vi "forma.vi"(5 "Input param":T1, 7 "GradFilePath":path caption="Градуировкиа:") -> ()   [LabVIEW 2010]
uses:
  <vilib>/Utility/config.llb/Read Key (Path).vi
  <vilib>/Utility/config.llb/Read Key (I32).vi
  <vilib>/Utility/config.llb/Write Key (I32).vi
  <vilib>/Utility/config.llb/NI_LVConfig.lvlib
panel:
  in  "Tab Control":T2(tab)
  in  "Channels":bool[](array[boolean]) caption="Каналы"
  in  "Sensors":string(combo) caption="Датчики:"
  in  "Conditions":string(combo) caption="Напряжение кВ:"
  in  "TesterName":string(combo) caption="Испытатель:"
  in  "Description":string(combo) caption="Измерение ЧР в:"
  out "ADCNum":string="Корона-20 № 11 АЦП 496" caption="Измеритель:"
  out "RepDate":string="2:23:15 24.11.2014" caption="Дата:"
  out "ObjName":string="Трансформатор № 1089-23" caption="Объект:"
  in  "RepNum":string="000012-03-2014.11.24" caption="Протокол номер:"
  in  "Concl":string="Заключение: " caption="Заключение"
  in  "CreateRepBtn":bool caption="Создать отчет"
  in  "ExitBtn":bool caption="Выйти"
  out "N(Q)":cluster{"x0":dbl, "dx":dbl, "y":sgl[][]}(graph) caption="Гистограмма N (Q)"
  out "Q(fi)":cluster{"x0":dbl, "dx":dbl, "y":sgl[][]}(graph) caption="Распределение @ ЧР по Фазе"
  out "Зависимость токов ЧР от I(R)":cluster{"x0":dbl, "dx":dbl, "y":sgl[][]}(graph) caption="Зависимость токов ЧР от коэффициента стационарности R"
  out "Q(R)":cluster{"x0":dbl, "dx":dbl, "y":sgl[][]}(graph) caption="Зависимость Q ЧР от коэффициента стационарности R"
  # "К1               К2               К3                К4"
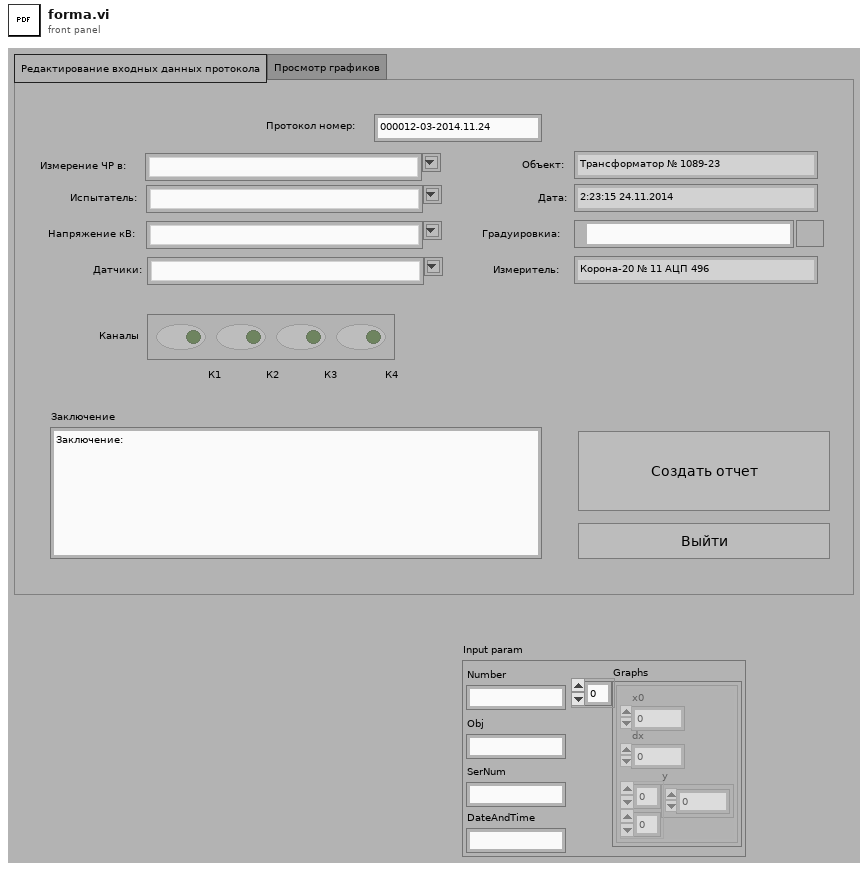
[diagram p1: front panel]
types:
  T1 = cluster{"Number":string, "Obj":string, "SerNum":string, "Graphs":cluster{"x0":dbl, "dx":dbl, "y":sgl[][]}[], "DateAndTime":string}
  T2 = enum32{"Редактирование входных данных протокола", "Просмотр графиков"}
  T3 = typedef "NI_LVConfig.lvlib/Config Data RefNum.ctl" = refnum<k1>
  T4 = cluster{"RepNum":string, "Description":string, "TesterName":string, "Conditions":string, "Sensors":string, "ObjName":string, string, string, "ADCNum":string, "Concl":string, "date/time string":string, "Channels":bool[], sgl[][]}
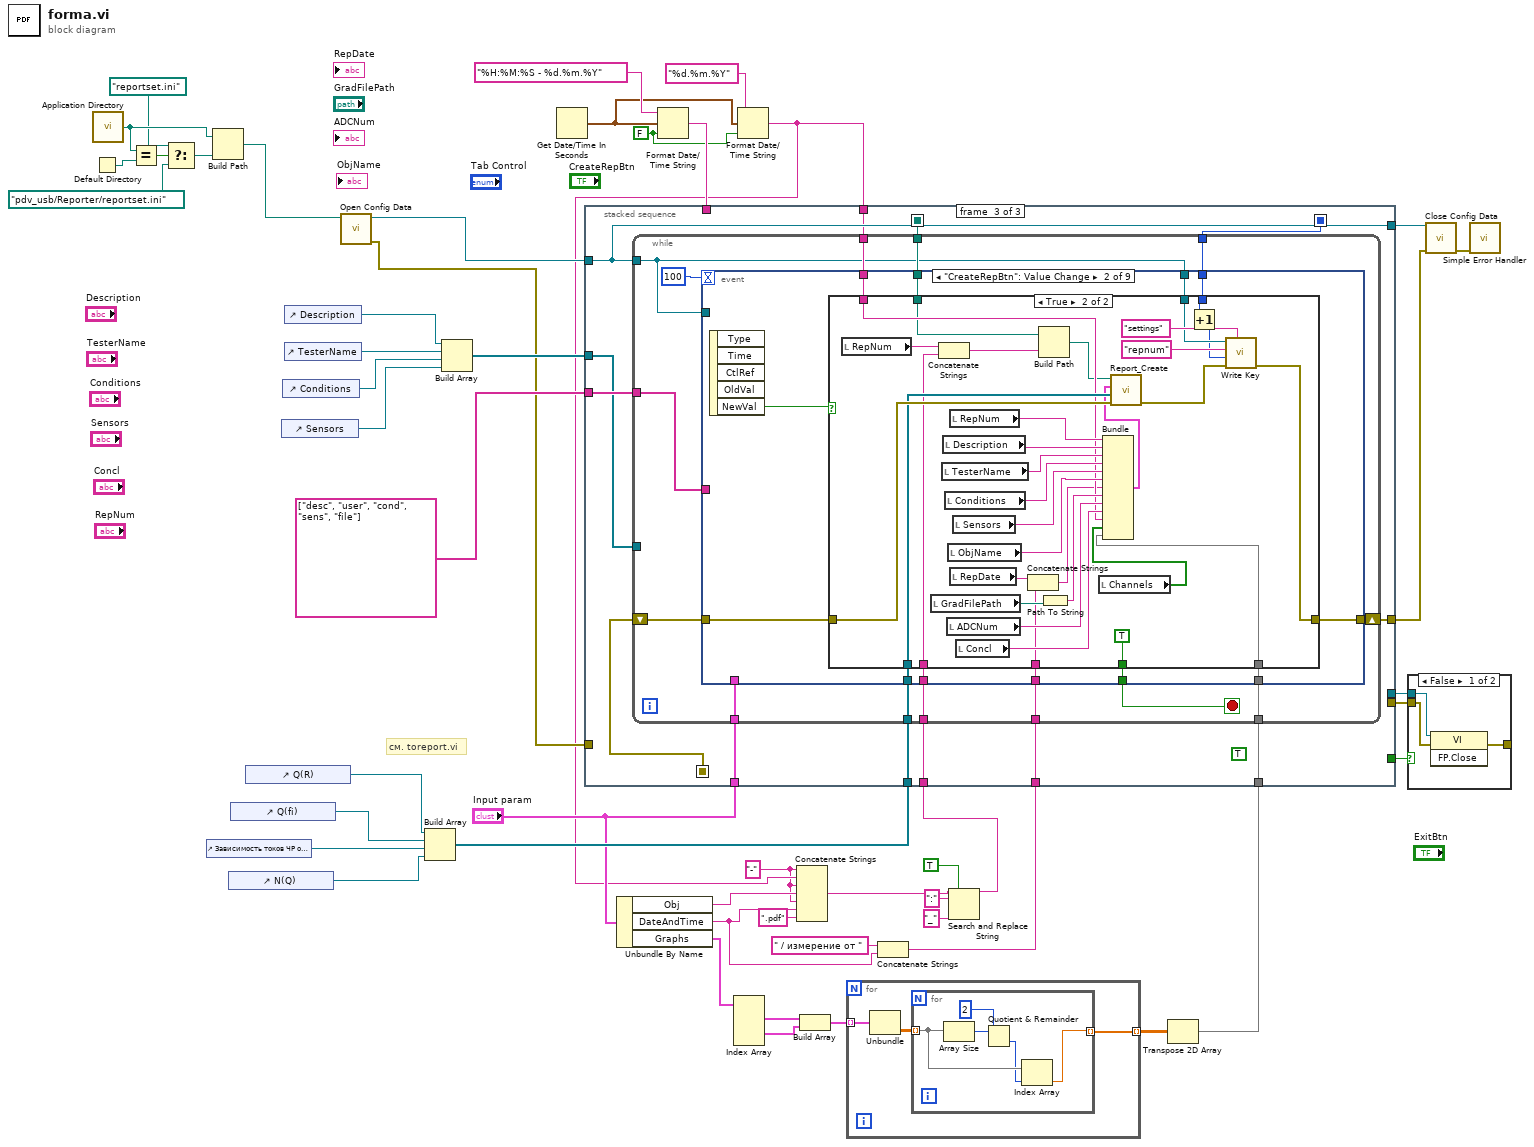
[diagram p0: block diagram]
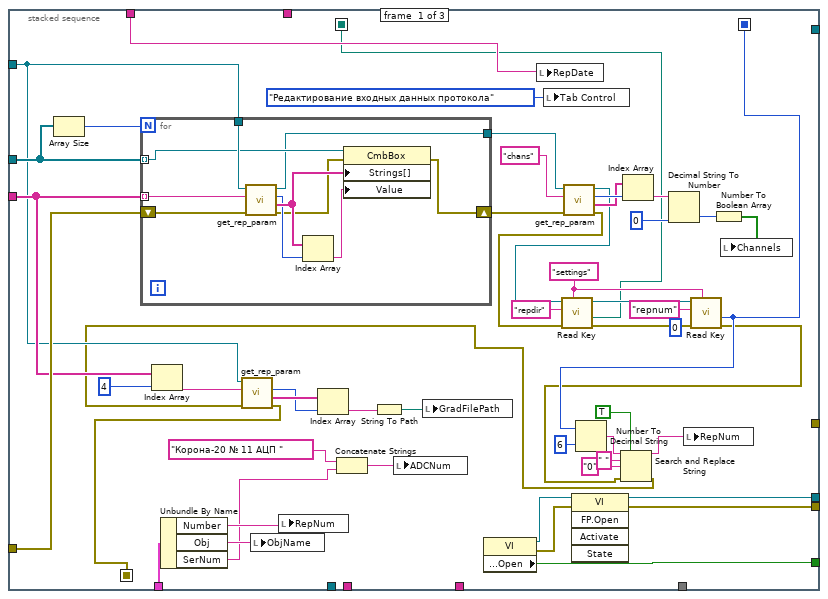
[diagram p3: hidden frame]
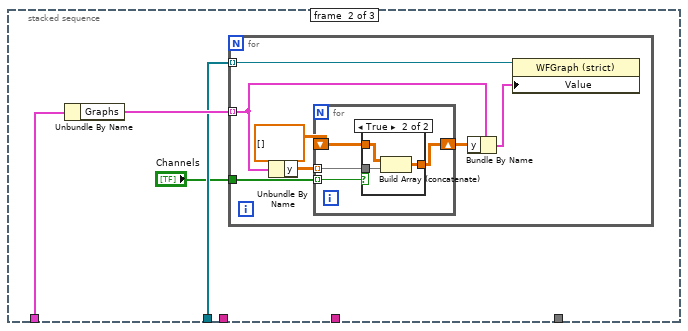
[diagram p4: hidden frame]
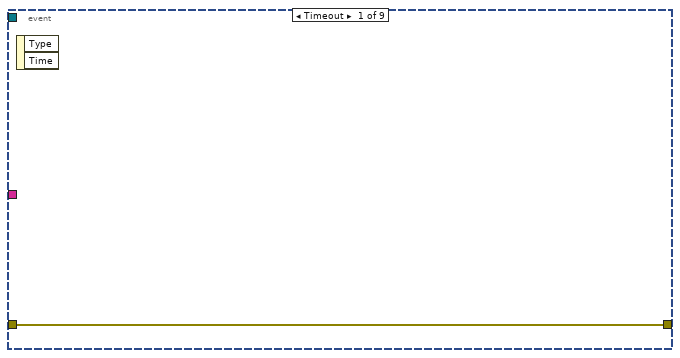
[diagram p6: hidden frame]
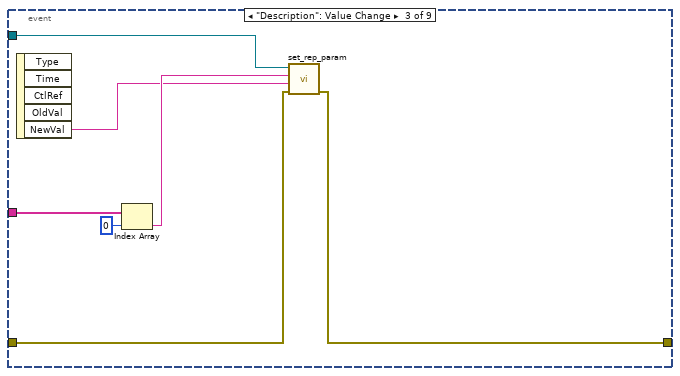
[diagram p8: hidden frame]
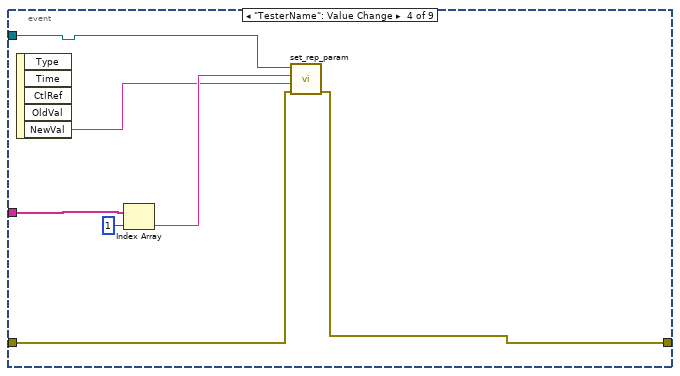
[diagram p9: hidden frame]
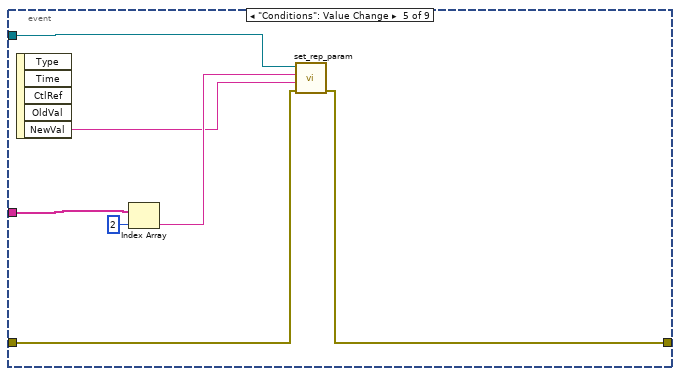
[diagram p10: hidden frame]
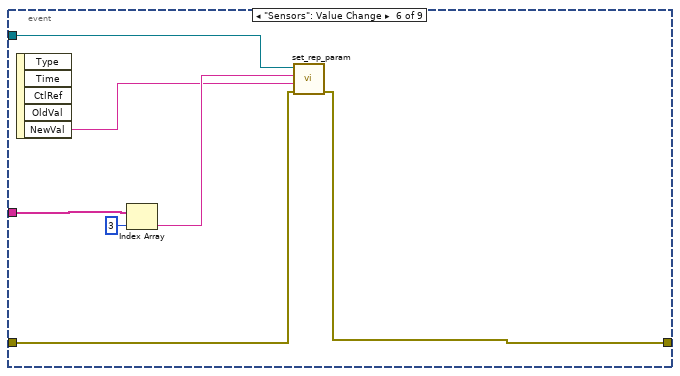
[diagram p11: hidden frame]
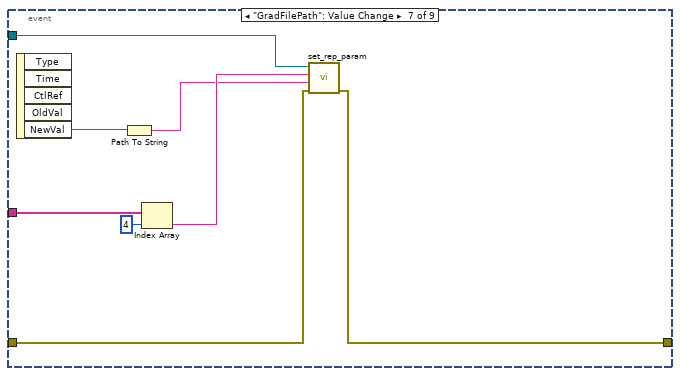
[diagram p12: hidden frame]
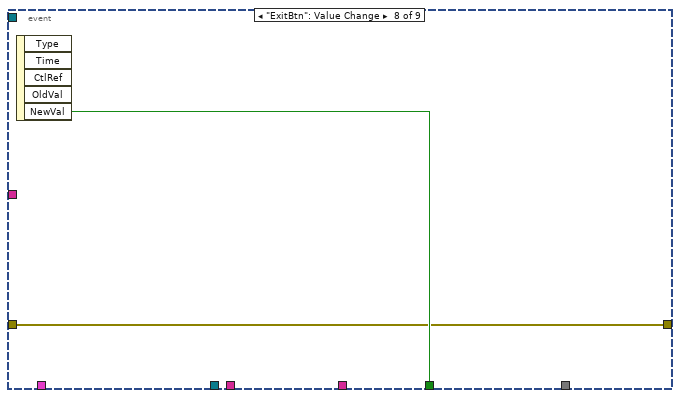
[diagram p13: hidden frame]
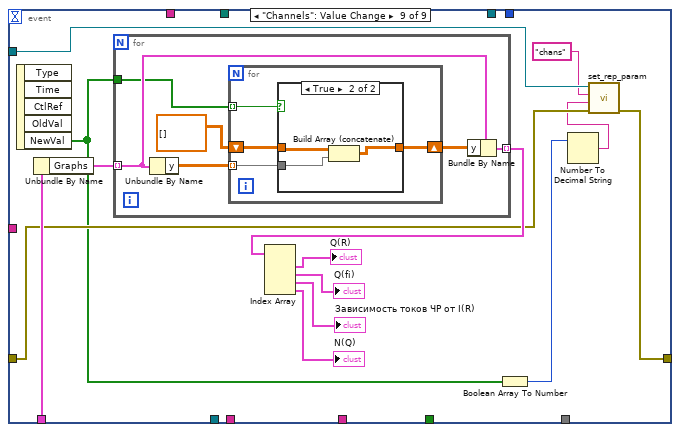
[diagram p14: hidden frame]
diagram:
  w16 = "-" ("string")
  w19 = FALSE ("UTC format")
  # "см. toreport.vi"
  n1 = Default Directory() -> (w28:path)
  n2 = call <vilib>:"Application Directory.vi"() -> ("Application Directory"=w27:path)
  n3 = Equal?(x=w27, y=w28) -> (x = y?=w26:bool)
  n4 = Select(t=path "reportset.ini" ("configuration file path"), s=w26, f=path "pdv_usb/Reporter/reportset.ini" ("configuration file path")) -> (s? t:f=w24:path)
  n5 = control-ref of="Зависимость токов ЧР от I(R)"() -> (w39:refnum<vi>)
  n6 = Build Path(base path=w27, name or relative path=w24) -> (appended path=w29:path)
  n7 = control-ref of="N(Q)"() -> (w38:refnum<vi>)
  n8 = control-ref of="Q(fi)"() -> (w40:refnum<vi>)
  n9 = control-ref of="Q(R)"() -> (w37:refnum<vi>)
  n10 = control-ref of="Sensors"() -> (w47:refnum<vi>)
  n11 = control-ref of="Conditions"() -> (w48:refnum<vi>)
  n12 = control-ref of="Description"() -> (w50:refnum<vi>)
  n13 = control-ref of="TesterName"() -> (w49:refnum<vi>)
  n14 = call <vilib>:"Open Config Data.vi"("configuration file path"=w29) -> ("error out"=w43:errorcluster, "refnum"=w44:T3)  [unwired: 8 in, 1 out]
  n15 = Build Array(w37, w40, w39, w38) -> (w36:refnum<vi>[])
  n16 = Build Array(w50, w49, w48, w47) -> (w46:refnum<vi>[])
  n17 = Get Date/Time In Seconds() -> (seconds since 1Jan1904=w20:timestamp)
  n18 = Unbundle By Name("Input param") -> ("Obj"=w17:string, "DateAndTime"=w13:string, "Graphs"=w6:cluster{"x0":dbl, "dx":dbl, "y":sgl[][]}[])
  n19 = Format Date/Time String(time format string (%c)="%H:%M:%S - %d.%m.%Y", seconds (now)=w20, UTC format=w19) -> (date/time string=w34:string)
  n20 = Index Array(array=w6) -> (element #1=w5:cluster{"x0":dbl, "dx":dbl, "y":sgl[][]}, element #3=w4:cluster{"x0":dbl, "dx":dbl, "y":sgl[][]})  [unwired: 4 in, 2 out]
  n21 = Format Date/Time String(time format string (%c)="%d.%m.%Y", seconds (now)=w20, UTC format=w19) -> (date/time string=w18:string)
  n22 = Concatenate Strings(w16, w18, w16, w17, w16, w13, ".pdf" ("string")) -> (w10:string)
  n23 = Build Array(w5, w4) -> (w3:cluster{"x0":dbl, "dx":dbl, "y":sgl[][]}[])
  n24 = for {
    tunnel: w3 -> [w53] mode=indexing
    tunnel: [w51] -> w2 mode=indexing
    n25 = Unbundle(w53) -> ("y"=w52:sgl[][])  [unwired: 2 out]
    n26 = for {
      tunnel: w52 -> [w56] mode=indexing
      tunnel: [w54] -> w51 mode=indexing
      n27 = Array Size(array=w56) -> (size(s)=w58:i32)
      n28 = Quotient & Remainder(x=w58, y=2) -> (floor(x/y)=w55:i32)  [unwired: 1 out]
      n29 = Index Array(array=w56, index=w55) -> (element=w54:sgl)
    }
  }
  n30 = Concatenate Strings(" / измерение от " ("string"), w13) -> (w12:string)
  n31 = Search and Replace String(replace all?=TRUE ("replace all? (F)"), input string=w10, search string=":", replace string="_" ("replace string (\"\")")) -> (result string=w9:string)  [unwired: 4 in, 3 out]
  n32 = Transpose 2D Array(2D array=w2) -> (transposed array=w1:sgl[][])
  n33 = stacked-sequence {
    seq-local: [w107 _ _] -> [_ _ w152]
    seq-local: [w59 _ _] -> [_ _ w143]
    seq-local: [w69 _ _] -> [_ _ w142]
    tunnel: w46 -> [w108 _ w149]
    tunnel: string[] ["desc", "user", "cond", "sens", "file"] -> [w105 _ w150]
    tunnel: w44 -> [w104 _ w148]
    tunnel: w43 -> [w110 _ _]
    tunnel: [_ _ w151] -> w41
    tunnel: [_ _ w148] -> w42
    tunnel: w36 -> [_ w122 w147]
    tunnel: w34 -> [w96 _ _]
    tunnel: "Input param" -> [w95 w124 w146]
    tunnel: [w89 _ _] -> w33
    tunnel: [w68 _ _] -> w32
    tunnel: [w88 _ _] -> w30
    tunnel: w18 -> [_ _ w145]
    tunnel: w9 -> [_ _ w144]
    tunnel: w12 -> [_ _ w141]
    tunnel: w1 -> [_ _ w140]
    frame #0 {
      w74 = "settings" ("section")
      n34 = Array Size(array=w108) -> (size(s)=w109:i32)
      n35 = for {
        N: w109 -> [_]
        tunnel: w108 -> [w117] mode=indexing
        tunnel: w105 -> [w119] mode=indexing
        tunnel: w104 -> [w120]
        shift-right: [w112] -> w85
        shift-left: w110 -> [w118]
        tunnel: [w111] -> w87
        n36 = call "get_rep_param.vi"("error in (no error)"=w118, "param_name"=w119, "refnum"=w120) -> ("error out"=w113:errorcluster, "list"=w116:string[], "default"=w115:i32, "refnum out"=w111:T3)  [unwired: 1 in]
        n37 = Index Array(array=w116, index=w115) -> (element=w114:string)
        n38 = property class="CmbBox"(reference=w117, error in=w113, "Strings[]"=w116, "Value"=w114) -> (error out=w112:errorcluster)  [unwired: 1 out]
      }
      n39 = Index Array(array=w105, index=4) -> (element=w103:string)
      n40 = Unbundle By Name(w95) -> ("Number"=w94:string, "Obj"=w93:string, "SerNum"=w92:string)
      n41 = local write "ObjName"(w93) -> ()
      n42 = local write "RepNum"(w94) -> ()
      n43 = Concatenate Strings("Корона-20 № 11 АЦП " ("time format string (%c)"), w92) -> (w97:string)
      n44 = local write "ADCNum"(w97) -> ()
      n45 = property class="VI"() -> (reference out=w91:refnum<vi>, error out=w90:errorcluster, "Front Panel.Open"=w89:bool)  [unwired: 2 in]
      n46 = local write "RepDate"(w96) -> ()
      n47 = local write "Tab Control"(T2."Редактирование входных данных протокола" ("Tab Control")) -> ()
      n48 = call "get_rep_param.vi"("error in (no error)"=w85, "param_name"="chans", "refnum"=w87) -> ("error out"=w78:errorcluster, "list"=w83:string[], "default"=w84:i32, "refnum out"=w76:T3)  [unwired: 1 in]
      n49 = call-poly <vilib>:"Read Key.vi"("section"=w74, "error in (no error)"=w78, "key"="repdir", "refnum"=w76) -> ("error out"=w77:errorcluster, "value"=w59:path, "refnum out"=w75:T3)  [unwired: 4 in, 1 out]
      n50 = invoke class="VI" method="FP.Open"(reference=w91, error in=w90) -> (reference out=w88:refnum<vi>, error out=w68:errorcluster)  [unwired: 3 in, 3 out]
      n51 = Index Array(array=w83, index=w84) -> (element=w82:string)
      n52 = Decimal String To Number(string=w82, default (0L)=u8 0) -> (number=w80:u8)  [unwired: 1 in, 1 out]
      n53 = call-poly <vilib>:"Read Key.vi"("section"=w74, "error in (no error)"=w77, "default value"=0, "key"="repnum", "refnum"=w75) -> ("error out"=w61:errorcluster, "value"=w69:i32)  [unwired: 3 in, 2 out]
      n54 = Number To Decimal String(number=w69, width (-)=i16 6) -> (decimal integer string=w65:string)
      n55 = Search and Replace String(replace all?=TRUE ("replace all? (F)"), input string=w65, search string=" ", replace string="0" ("replace string (\"\")"), error in=w61) -> (result string=w64:string, error out=w60:errorcluster)  [unwired: 3 in, 2 out]
      n56 = call "get_rep_param.vi"("error in (no error)"=w60, "param_name"=w103, "refnum"=w104) -> ("error out"=w107:errorcluster, "list"=w102:string[], "default"=w101:i32)  [unwired: 1 in, 1 out]
      n57 = Index Array(array=w102, index=w101) -> (element=w100:string)
      n58 = String To Path(string=w100) -> (path=w99:path)
      n59 = local write "GradFilePath"(w99) -> ()
      n60 = local write "RepNum"(w64) -> ()
      n61 = Number To Boolean Array(number=w80) -> (Boolean array=w79:bool[])
      n62 = local write "Channels"(w79) -> ()
    }
    frame #1 {
      n63 = Unbundle By Name(w124) -> ("Graphs"=w123:cluster{"x0":dbl, "dx":dbl, "y":sgl[][]}[])
      n64 = for {
        tunnel: w123 -> [w127] mode=indexing
        tunnel: w122 -> [w131] mode=indexing
        tunnel: "Channels" -> [w130]
        n65 = Unbundle By Name(w127) -> ("y"=w129:sgl[][])
        n66 = for {
          tunnel: w130 -> [w132] mode=indexing
          tunnel: w129 -> [w135] mode=indexing
          shift-right: [w134] -> w125
          shift-left: sgl[][] [] -> [w133]
          n67 = case shown="True" w132 {
            tunnel: w135 -> [_ w139]
            tunnel: [w136 w138] -> w134
            tunnel: w133 -> [w136 w137]
            frame False {
            }
            frame True {
              n68 = Build Array (concatenate)(w137, w139) -> (w138:sgl[][])
            }
          }
        }
        n69 = Bundle By Name(cluster=w127, "y"=w125) -> (w126:cluster{"x0":dbl, "dx":dbl, "y":sgl[][]})
        n70 = property class="WFGraph (strict)"(reference=w131, "Value"=w126) -> ()  [unwired: 1 in, 2 out]
      }
    }
    frame #2 {
      (unwired) TRUE
      n71 = while {
        shift-right: [w164] -> w151
        shift-left: w152 -> [w165]
        tunnel: w148 -> [w156]
        tunnel: w150 -> [w163]
        tunnel: w149 -> [_]
        tunnel: w147 -> [w161]
        tunnel: w146 -> [w160]
        tunnel: w145 -> [w159]
        tunnel: w144 -> [w158]
        tunnel: w143 -> [w157]
        tunnel: w142 -> [w155]
        tunnel: w141 -> [w154]
        tunnel: w140 -> [w153]
        stop <- w166 stop-if-true
        n72 = event shown="[1] \"CreateRepBtn\": Value Change" {
          selector: _ -> [_ _ _ _ _ _ _ _ _]
          dyn-events: _ -> [_ _ _ _ _ _ _ _ _]
          timeout: 100 -> [_ _ _ _ _ _ _ _ _]
          tunnel: [_ w178 _ _ _ _ _ w250 _] -> w166
          tunnel: w165 -> [w167 w176 w218 w222 w230 w237 w244 w249 w255]
          tunnel: [w167 w177 w217 w223 w229 w236 w243 w249 w254] -> w164
          tunnel: w156 -> [_ _ w219 w224 w231 w238 w246 _ w257]
          tunnel: w163 -> [_ _ w216 w221 w228 w235 w245 _ _]
          tunnel: w161 -> [_ w175 _ _ _ _ _ _ _]
          tunnel: w160 -> [_ _ _ _ _ _ _ _ w258]
          tunnel: w159 -> [_ w174 _ _ _ _ _ _ _]
          tunnel: w158 -> [_ w173 _ _ _ _ _ _ _]
          tunnel: w157 -> [_ w172 _ _ _ _ _ _ _]
          tunnel: w156 -> [_ w171 _ _ _ _ _ _ _]
          tunnel: w155 -> [_ w170 _ _ _ _ _ _ _]
          tunnel: w154 -> [_ w169 _ _ _ _ _ _ _]
          tunnel: w153 -> [_ w168 _ _ _ _ _ _ _]
          event Timeout {
            n73 = event-data() -> ()  [unwired: 1 in, 2 out]
          }
          event "CreateRepBtn": Value Change {
            n74 = event-data() -> ("NewVal"=w179:bool)  [unwired: 1 in, 4 out]
            n75 = case shown="True" w179 {
              tunnel: [_ TRUE] -> w178
              tunnel: [w180 w192] -> w177
              tunnel: w176 -> [w180 w211]
              tunnel: w175 -> [_ w210]
              tunnel: w174 -> [_ w197]
              tunnel: w173 -> [_ w195]
              tunnel: w172 -> [_ w184]
              tunnel: w171 -> [_ w188]
              tunnel: w170 -> [_ w189]
              tunnel: w169 -> [_ w185]
              tunnel: w168 -> [_ w181]
              frame False {
              }
              frame True {
                n76 = local read "RepNum"() -> (w196:string)
                n77 = local read "GradFilePath"() -> (w199:path)
                n78 = Concatenate Strings(w196, w195) -> (w194:string)
                n79 = local read "TesterName"() -> (w207:string)
                n80 = local read "Description"() -> (w208:string)
                n81 = local read "Conditions"() -> (w206:string)
                n82 = local read "ADCNum"() -> (w202:string)
                n83 = local read "ObjName"() -> (w204:string)
                n84 = local read "RepNum"() -> (w209:string)
                n85 = local read "RepDate"() -> (w203:string)
                n86 = local read "Sensors"() -> (w205:string)
                n87 = local read "Concl"() -> (w201:string)
                n88 = Concatenate Strings(w203, w185) -> (w186:string)
                n89 = Build Path(base path=w184, name or relative path=w194) -> (appended path=w183:path)
                n90 = Path To String(path=w199) -> (string=w198:string)
                n91 = local read "Channels"() -> (w182:bool[])
                n92 = Bundle("RepNum"=w209, "Description"=w208, "TesterName"=w207, "Conditions"=w206, "Sensors"=w205, "ObjName"=w204, w186, w198, "ADCNum"=w202, "Concl"=w201, "date/time string"=w197, "Channels"=w182, w181) -> (w200:T4)  [unwired: 1 in]
                n93 = call "Report_Create.vi"("error in (no error)"=w211, "appended array 2"=w210, "output cluster"=w200, "Save Filename"=w183) -> ("error out"=w193:errorcluster)  [unwired: 7 in]
                n94 = Increment(x=w189) -> (x+1=w187:i32)
                n95 = call-poly <vilib>:"Write Key.vi"("section"="settings", "error in (no error)"=w193, "value"=w187, "key"="repnum", "refnum"=w188) -> ("error out"=w192:errorcluster)  [unwired: 4 in, 2 out]
              }
            }
          }
          event "Description": Value Change {
            n96 = event-data() -> ("NewVal"=w213:string)  [unwired: 1 in, 4 out]
            n97 = Index Array(array=w216, index=0) -> (element=w215:string)
            n98 = call "set_rep_param.vi"("error in (no error)"=w218, "par_val"=w213, "param_name"=w215, "refnum"=w219) -> ("error out"=w217:errorcluster)  [unwired: 2 in, 1 out]
          }
          event "TesterName": Value Change {
            n99 = event-data() -> ("NewVal"=w220:string)  [unwired: 1 in, 4 out]
            n100 = Index Array(array=w221, index=1) -> (element=w225:string)
            n101 = call "set_rep_param.vi"("error in (no error)"=w222, "par_val"=w220, "param_name"=w225, "refnum"=w224) -> ("error out"=w223:errorcluster)  [unwired: 2 in, 1 out]
          }
          event "Conditions": Value Change {
            n102 = event-data() -> ("NewVal"=w227:string)  [unwired: 1 in, 4 out]
            n103 = Index Array(array=w228, index=2) -> (element=w232:string)
            n104 = call "set_rep_param.vi"("error in (no error)"=w230, "par_val"=w227, "param_name"=w232, "refnum"=w231) -> ("error out"=w229:errorcluster)  [unwired: 2 in, 1 out]
          }
          event "Sensors": Value Change {
            n105 = event-data() -> ("NewVal"=w234:string)  [unwired: 1 in, 4 out]
            n106 = Index Array(array=w235, index=3) -> (element=w239:string)
            n107 = call "set_rep_param.vi"("error in (no error)"=w237, "par_val"=w234, "param_name"=w239, "refnum"=w238) -> ("error out"=w236:errorcluster)  [unwired: 2 in, 1 out]
          }
          event "GradFilePath": Value Change {
            n108 = event-data() -> ("NewVal"=w242:path)  [unwired: 1 in, 4 out]
            n109 = Path To String(path=w242) -> (string=w241:string)
            n110 = Index Array(array=w245, index=4) -> (element=w247:string)
            n111 = call "set_rep_param.vi"("error in (no error)"=w244, "par_val"=w241, "param_name"=w247, "refnum"=w246) -> ("error out"=w243:errorcluster)  [unwired: 2 in, 1 out]
          }
          event "ExitBtn": Value Change {
            n112 = event-data() -> ("NewVal"=w250:bool)  [unwired: 1 in, 4 out]
          }
          event "Channels": Value Change {
            n113 = event-data() -> ("NewVal"=w252:bool[])  [unwired: 1 in, 4 out]
            n114 = Unbundle By Name(w258) -> ("Graphs"=w264:cluster{"x0":dbl, "dx":dbl, "y":sgl[][]}[])
            n115 = for {
              tunnel: w252 -> [w265]
              tunnel: w264 -> [w270] mode=indexing
              tunnel: [w269] -> w263 mode=indexing
              n116 = Unbundle By Name(w270) -> ("y"=w267:sgl[][])
              n117 = for {
                shift-right: [w273] -> w268
                shift-left: sgl[][] [] -> [w274]
                tunnel: w265 -> [w272] mode=indexing
                tunnel: w267 -> [w271] mode=indexing
                n118 = case shown="True" w272 {
                  tunnel: w274 -> [w275 w276]
                  tunnel: [w275 w277] -> w273
                  tunnel: w271 -> [_ w278]
                  frame False {
                  }
                  frame True {
                    n119 = Build Array (concatenate)(w276, w278) -> (w277:sgl[][])
                  }
                }
              }
              n120 = Bundle By Name(cluster=w270, "y"=w268) -> (w269:cluster{"x0":dbl, "dx":dbl, "y":sgl[][]})
            }
            n121 = Index Array(array=w263) -> (element #1=→"Q(R)":cluster{"x0":dbl, "dx":dbl, "y":sgl[][]}, element #2=→"Q(fi)":cluster{"x0":dbl, "dx":dbl, "y":sgl[][]}, element #3=→"Зависимость токов ЧР от I(R)":cluster{"x0":dbl, "dx":dbl, "y":sgl[][]}, element #4=→"N(Q)":cluster{"x0":dbl, "dx":dbl, "y":sgl[][]})  [unwired: 4 in]
            n122 = Boolean Array To Number(Boolean array=w252) -> (number=w251:u32)
            n123 = Number To Decimal String(number=w251) -> (decimal integer string=w253:string)  [unwired: 1 in]
            n124 = call "set_rep_param.vi"("error in (no error)"=w255, "par_val"=w253, "param_name"="chans", "refnum"=w257) -> ("error out"=w254:errorcluster)  [unwired: 2 in, 1 out]
          }
        }
      }
    }
  }
  n125 = case shown="False" w33 {
    tunnel: w32 -> [w281 _]
    tunnel: [w280 _] -> _
    tunnel: w30 -> [w279 _]
    frame False {
      n126 = invoke class="VI" method="FP.Close"(reference=w279, error in=w281) -> (error out=w280:errorcluster)  [unwired: 1 in, 2 out]
    }
    frame True {
    }
  }
  n127 = call <vilib>:"Close Config Data.vi"("error in (no error)"=w41, "refnum"=w42) -> ("error out"=w31:errorcluster)  [unwired: 8 in, 1 out]
  n128 = call <vilib>:"Simple Error Handler.vi"("error in (no error)"=w31) -> ()  [unwired: 4 in, 5 out]
